vi "TETRIX Motor Move_HT_myRIO_ver2.vi"(0 "error in (no error)":errorcluster, 1 "Select Channel":string(combo)="Motor 1", 2 "Controller Daisy Chain Position: 1 - 4":u8=1 min=1 max=4, 3 "Encoder Target: 360 = 1 motor shaft revolution":i32, 4 "Reverse? : T or F":bool, 6 "Control Mode":string(combo)="Power Only", 7 "Port":enum16{"Port A", "Port B", ""}(ring), 8 "Power (-100 to 100)\n0 = Stop/Brake\n-128 = Stop/Coast":i8(slide) scale=-100.0..100.0) -> (5 "error out":errorcluster)   [LabVIEW 2015]
uses:
  <vilib>/myRIO/Instrument Drivers/Onboard IO/I2C/typedefs/I2C User Configuration.ctl
  <vilib>/myRIO/Instrument Drivers/Onboard IO/I2C/typedefs/I2C Transfer Rate.ctl
  <vilib>/myRIO/Instrument Drivers/Onboard IO/I2C/typedefs/I2C Reference.ctl
  <vilib>/myRIO/Common/Instrument Driver Framework/Utilities/typedefs/myRIO Generic Hardware Reference.ctl
  <vilib>/myRIO/Common/Instrument Driver Framework/Utilities/typedefs/Hardware Version Enum.ctl
  <vilib>/myRIO/Common/Instrument Driver Framework/Utilities/typedefs/myRIO v1.0 Reference.ctl
  <vilib>/myRIO/Common/Instrument Driver Framework/Utilities/typedefs/Generic FPGA Reference.ctl
  <vilib>/myRIO/Common/Instrument Driver Framework/myRIO v1.0/I2C/typedefs/I2C Channels Enum.ctl
  <vilib>/myRIO/Instrument Drivers/Onboard IO/I2C/typedefs/I2C Configuration.ctl
  <vilib>/userdefined/High Color/nirio_resource_hc.ctl
  <vilib>/myRIO/Common/Instrument Driver Framework/Utilities/vis/Is FPGA Ref Available.vi
  <vilib>/myRIO/Common/Instrument Driver Framework/myRIO v1.0/I2C/vis/myRIO v1.1 Open I2C.vi
  <vilib>/myRIO/Instrument Drivers/Onboard IO/I2C/vis/Configure.vi
  <vilib>/myRIO/Instrument Drivers/Onboard IO/I2C/vis/Write.vi
  <vilib>/myRIO/Common/Instrument Driver Framework/Utilities/vis/Validate Channels.vi
  <vilib>/myRIO/Common/Instrument Driver Framework/myRIO v1.0/I2C/vis/myRIO v1.0 Reserve I2C.vi
  <vilib>/myRIO/Common/Instrument Driver Framework/myRIO v1.0/I2C/vis/myRIO v1.0 Build MUX Configuration I2C.vi
  <vilib>/myRIO/Common/Instrument Driver Framework/myRIO v1.0/Resource Manager/vis/myRIO v1.0 Reserve Channel List.vi
  <vilib>/myRIO/Common/Instrument Driver Framework/myRIO v1.0/Resource Manager/vis/myRIO v1.0 Create Configuration List.vi
  <vilib>/myRIO/Common/Instrument Driver Framework/myRIO v1.0/Resource Manager/vis/myRIO v1.0 Reserve Channel.vi
  <vilib>/myRIO/Common/Instrument Driver Framework/myRIO v1.0/Resource Manager/vis/myRIO v1.0 Unreserve Channel.vi
  <vilib>/myRIO/Common/Instrument Driver Framework/myRIO v1.0/Resource Manager/vis/myRIO v1.0 Build Mutex Name.vi
  <vilib>/Utility/VariantDataType/GetNumericInfo.vi
  <vilib>/Utility/error.llb/Error Cluster From Error Code.vi
  <vilib>/myRIO/Common/Instrument Driver Framework/myRIO v1.0/myRIO v1.1 Open.vi
  <vilib>/myRIO/Common/Instrument Driver Framework/Utilities/vis/IO Manager.vi
  <vilib>/myRIO/Common/Instrument Driver Framework/Utilities/vis/Configuration Manager.vi
  <vilib>/myRIO/Common/Instrument Driver Framework/myRIO v1.0/Resource Manager/vis/myRIO v1.0 Configure IO.vi
  <vilib>/myRIO/Common/Instrument Driver Framework/myRIO v1.0/myRIO v1.0 Close.vi
  <vilib>/myRIO/Common/Instrument Driver Framework/myRIO v1.0/I2C/vis/myRIO v1.0 Configure I2C.vi
  <vilib>/myRIO/Common/Instrument Driver Framework/myRIO v1.0/I2C/vis/myRIO v1.0 Write I2C.vi
  <vilib>/myRIO/Express VI/Onboard IO/I2C/I2C Express VI.xnode
  <vilib>/myRIO/Instrument Drivers/Onboard IO/I2C/vis/myRIO I2C Open.xnode
  <vilib>/myRIO/Instrument Drivers/Onboard IO/I2C/I2C.lvlib
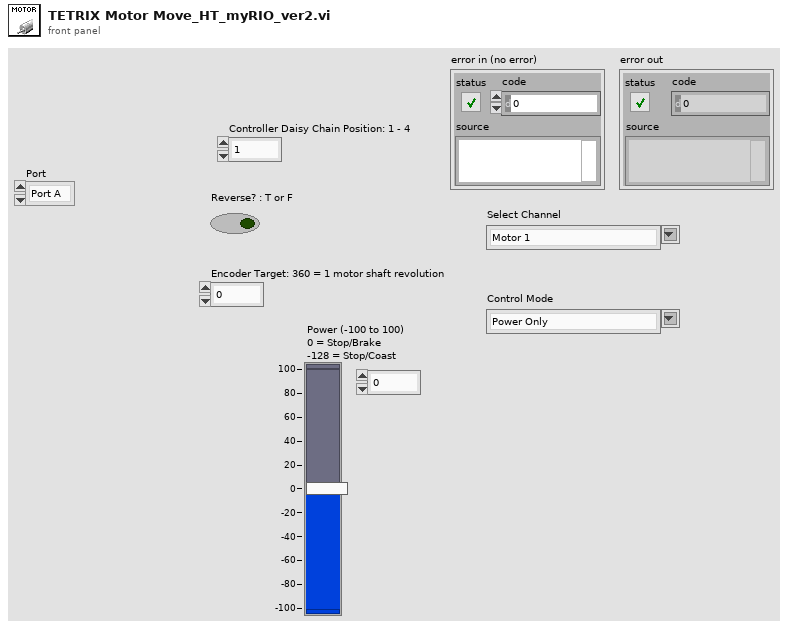
[diagram p1: front panel]
types:
  T1 = typedef "I2C.lvlib/I2C Reference.ctl" = cluster{"myRIO Reference":T2, "I2C Channels Enum":T6, "I2C Configuration":T7}
  T2 = typedef "myRIO Generic Hardware Reference.ctl" = cluster{"myRIO Model":T3, "myRIO Hardware Reference":T4}
  T3 = typedef "Hardware Version Enum.ctl" = enum16{"Unknown", "myRIO-1900", "myRIO-1950", "roboRIO"}
  T4 = typedef "myRIO v1.0 Reference.ctl" = cluster{"Generic FPGA Reference":T5, "Allow multiple opens":bool}
  T5 = typedef "Generic FPGA Reference.ctl" = refnum<k20>
  T6 = typedef "I2C Channels Enum.ctl" = enum16{"Not Connected", "A/I2C", "B/I2C", "I2C/I2C"}
  T7 = typedef "I2C.lvlib/I2C Configuration.ctl" = cluster{"I2C Transfer Rate":T8}
  T8 = typedef "I2C.lvlib/I2C Transfer Rate.ctl" = enum16{"Standard mode (100 kbps)", "Fast mode (400 kbps)"}
  T9 = typedef "I2C.lvlib/I2C User Configuration.ctl" = cluster{"I2C Transfer Rate":T8}
  T10 = typedef "nirio_resource_hc.ctl" = tag
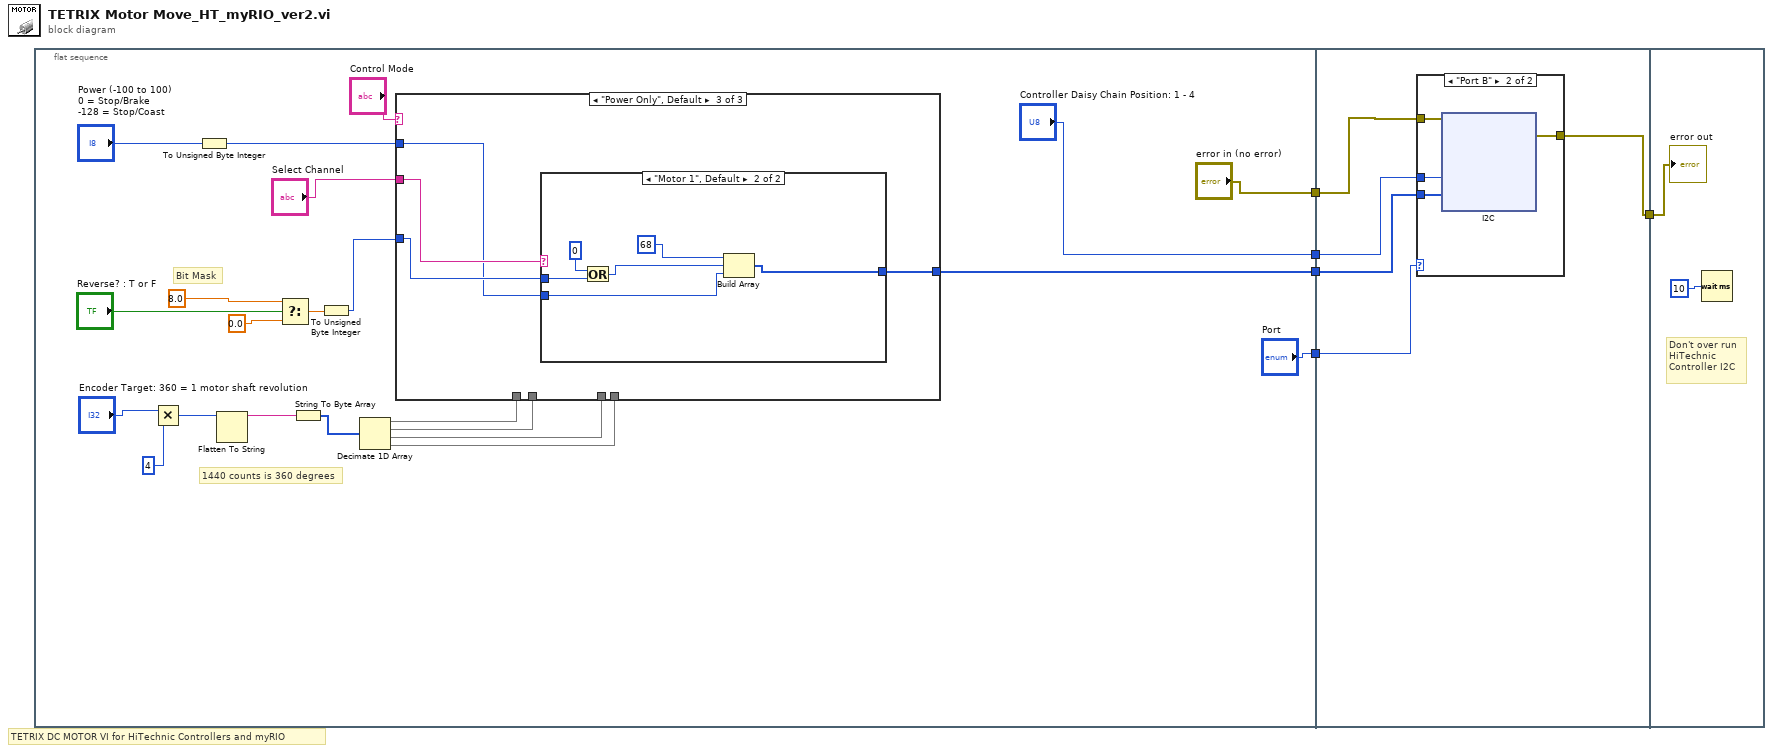
[diagram p0: block diagram]
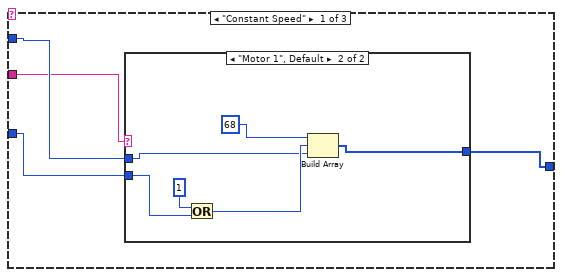
[diagram p2: hidden frame]
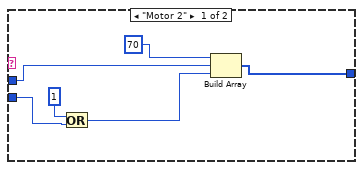
[diagram p3: hidden frame]
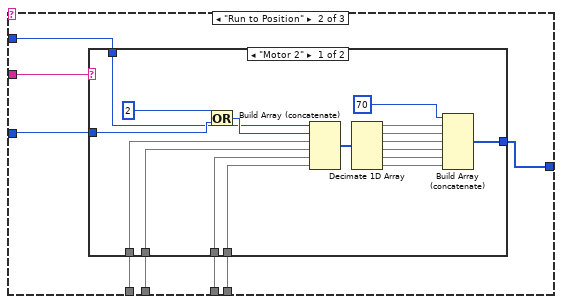
[diagram p4: hidden frame]
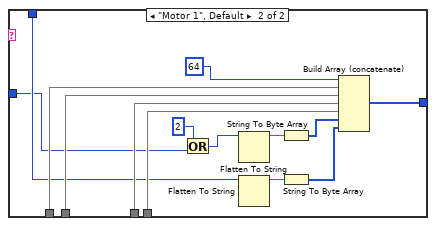
[diagram p5: hidden frame]
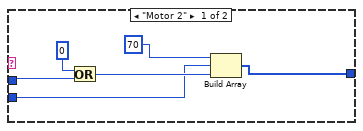
[diagram p6: hidden frame]
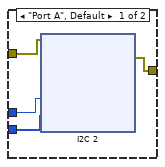
[diagram p7: hidden frame]
diagram:
  # "TETRIX DC MOTOR VI for HiTechnic Controllers and myRIO"
  n1 = flat-sequence {
    tunnel: ["Controller Daisy Chain Position: 1 - 4"] -> w5
    tunnel: [w16] -> w4
    tunnel: ["error in (no error)"] -> w3
    tunnel: ["Port"] -> w1
    tunnel: w5 -> [w103]
    tunnel: w4 -> [w102]
    tunnel: w3 -> [w101]
    tunnel: [w100] -> w2
    tunnel: w1 -> [w99]
    tunnel: w2 -> [w188]
    frame #0 {
      # "1440 counts is 360 degrees"
      # "Bit Mask"
      n2 = Multiply(x="Encoder Target: 360 = 1 motor shaft revolution", y=4) -> (x*y=w8:i32)
      n3 = To Unsigned Byte Integer(number="Power (-100 to 100)\n0 = Stop/Brake\n-128 = Stop/Coast") -> (unsigned 8bit integer=w18:u8)
      n4 = Flatten To String(anything=w8) -> (data string=w27:string)  [unwired: 3 in, 2 out]
      n5 = Select(t=8.0, s="Reverse? : T or F", f=0.0) -> (s? t:f=w23:dbl)
      n6 = String To Byte Array(string=w27) -> (unsigned byte array=w15:u8[])
      n7 = To Unsigned Byte Integer(number=w23) -> (unsigned 8bit integer=w19:u8)
      n8 = Decimate 1D Array(w15) -> (w14:u8[], w13:u8[], w12:u8[], w11:u8[])
      n9 = case shown="\"Power Only\", Default" "Control Mode" {
        tunnel: "Select Channel" -> [w28 w51 w86]
        tunnel: w19 -> [w30 w50 w85]
        tunnel: w18 -> [w31 w49 w84]
        tunnel: [w29 w48 w83] -> w16
        tunnel: w14 -> [_ w47 _]
        tunnel: w13 -> [_ w46 _]
        tunnel: w12 -> [_ w45 _]
        tunnel: w11 -> [_ w44 _]
        frame "Constant Speed" {
          n10 = case shown="\"Motor 1\", Default" w28 {
            tunnel: w31 -> [w33 w38]
            tunnel: w30 -> [w34 w40]
            tunnel: [w35 w41] -> w29
            frame "Motor 2" {
              n11 = Or(x=u8 1, y=w34) -> (x .or. y?=w32:u8)
              n12 = Build Array(u8 70, w33, w32) -> (w35:u8[])
            }
            frame "Motor 1", Default {
              n13 = Or(x=u8 1, y=w40) -> (x .or. y?=w39:u8)
              n14 = Build Array(u8 68, w39, w38) -> (w41:u8[])
            }
          }
        }
        frame "Run to Position" {
          n15 = case shown="\"Motor 2\"" w51 {
            tunnel: w50 -> [w58 w69]
            tunnel: w49 -> [w57 w72]
            tunnel: [w56 w80] -> w48
            tunnel: w47 -> [w55 w73]
            tunnel: w46 -> [w54 w74]
            tunnel: w45 -> [w53 w75]
            tunnel: w44 -> [w52 w76]
            frame "Motor 2" {
              n16 = Or(x=u8 2, y=w58) -> (x .or. y?=w59:u8)
              n17 = Build Array (concatenate)(w57, w59, w55, w54, w53, w52) -> (w68:u8[])
              n18 = Decimate 1D Array(w68) -> (w62:u8[], w63:u8[], w64:u8[], w65:u8[], w66:u8[], w67:u8[])
              n19 = Build Array (concatenate)(u8 70, w62, w63, w64, w65, w66, w67) -> (w56:u8[])
            }
            frame "Motor 1", Default {
              n20 = Or(x=u8 2, y=w69) -> (x .or. y?=w70:u8)
              n21 = Flatten To String(anything=w70) -> (data string=w81:string)  [unwired: 3 in, 2 out]
              n22 = Flatten To String(anything=w72) -> (data string=w82:string)  [unwired: 3 in, 2 out]
              n23 = String To Byte Array(string=w81) -> (unsigned byte array=w77:u8[])
              n24 = String To Byte Array(string=w82) -> (unsigned byte array=w78:u8[])
              n25 = Build Array (concatenate)(u8 64, w73, w74, w75, w76, w77, w78) -> (w80:u8[])
            }
          }
        }
        frame "Power Only", Default {
          n26 = case shown="\"Motor 1\", Default" w86 {
            tunnel: w85 -> [w90 w96]
            tunnel: w84 -> [w87 w93]
            tunnel: [w89 w95] -> w83
            frame "Motor 2" {
              n27 = Or(x=u8 0, y=w90) -> (x .or. y?=w88:u8)
              n28 = Build Array(u8 70, w87, w88) -> (w89:u8[])
            }
            frame "Motor 1", Default {
              n29 = Or(x=u8 0, y=w96) -> (x .or. y?=w94:u8)
              n30 = Build Array(u8 68, w94, w93) -> (w95:u8[])
            }
          }
        }
      }
    }
    frame #1 {
      n31 = case shown="\"Port B\"" w99 {
        tunnel: w103 -> [w105 w149]
        tunnel: w102 -> [w104 w148]
        tunnel: w101 -> [w107 w147]
        tunnel: [w106 w146] -> w100
        frame "Port A", Default {
          n32 = xnode "I2C 2"("Slave Address (7-bit)"=w105, "Bytes to Write"=w104, "error in (no error)"=w107) -> ("error out"=w106:errorcluster)
        }
        frame "Port B" {
          n33 = xnode "I2C"("Slave Address (7-bit)"=w149, "Bytes to Write"=w148, "error in (no error)"=w147) -> ("error out"=w146:errorcluster)
        }
      }
    }
    frame #2 {
      # "Don't over run\nHiTechnic\nController I2C"
      n34 = Wait (ms)(milliseconds to wait=u32 10) -> ()  [unwired: 1 out]
      "error out" <- w188
    }
  }
